vi "Main.vi"(11 "Module Admin":refnum<class "Delacor_lib_QMH_Module Admin.lvclass">) -> ()   [LabVIEW 2022 SP3, in "Motor.lvlib"]
doc: "This template is based off of the Queued Message Handler design pattern and the Queued Message Handler project template that ships with LabVIEW.\n\nThe main difference is that the queue is private to this module and communication between modules is performed via Broadcast and Request events.\n\nRequest events are wrapped in public API methods and are handled in the Event Handling Loop (EHL) of this VI. Any module can register for Broadcast events sent by this module. The EHL generates messages based on user interface actions.\n\nThe Message Handling Loop (MHL) processes messages generated by the EHL, or by other messages. The messages are string values, so new messages can be added easily to the Message Cases case structure in the MHL. Each message cluster can also provide an optional value for Message Data, which is a variant that can be converted to whatever message-specific data is required.\n_____\nBased on DQMH Project Template 7.0.1.1316."
uses:
  Motor.lvlib
  <vilib>/Delacor/Delacor QMH/Libraries/Module Admin_class/Delacor_lib_QMH_Module Admin.lvclass
  Module Data--cluster.ctl
  <vilib>/Delacor/Delacor QMH/Libraries/Message Queue_class/Delacor_lib_QMH_Message Queue.lvclass/Delacor_lib_QMH_Message Queue.ctl
  Stop Argument--cluster.ctl
  <vilib>/Delacor/Delacor QMH/Libraries/Module Admin_class/Delacor_lib_QMH_Module Admin.lvclass/Delacor_lib_QMH_Module Admin.ctl
  Moving Argument--cluster.ctl
  <vilib>/Utility/miscctls.llb/LVPointTypeDef.ctl
  <vilib>/MakerHub/LINX/Private/Type Defs/LINX Ref.ctl
  <vilib>/MakerHub/LINX/Private/Type Defs/Platform.ctl
  <vilib>/MakerHub/LINX/Private/Type Defs/Interface.ctl
  <vilib>/MakerHub/LINX/Private/Device/Type Defs/LINX Device Config.ctl
  <vilib>/MakerHub/LINX/Private/Device/Type Defs/TCP Config.ctl
  <vilib>/MakerHub/LINX/Private/Device/Type Defs/Channels.ctl
  Motorshield/DCMotor/DCMotor.lvclass
  <vilib>/Delacor/Delacor QMH/Libraries/Message Queue_class/Delacor_lib_QMH_Enqueue Message (Single).vi
  <vilib>/Delacor/Delacor QMH/Libraries/Module Admin_class/Delacor_lib_QMH_Get External Launch.vi
  <vilib>/Delacor/Delacor QMH/Libraries/Message Queue_class/Delacor_lib_QMH_Message Queue.lvclass
  <vilib>/MakerHub/LINX/LMH-LINX.lvlib
  <vilib>/MakerHub/LINX/Private/Device/Device.lvlib
  BME680/BME680_dqmh.lvlib
panel:
  out "error out":errorcluster
  out "Status":string
  in  "Simulate MHL Error":bool
  in  "Simulate EHL Error":bool
  # "Other processes communicate with this Module via its Public API (wrappers for its Request Events).\n\nThis Module communicates with other processes via its Broadcast Events.\nAny process that wants to receive these messages can register for this module's Broadcast events."
  # "This template is for the DQMH framework. See the block diagram for more information on how to use this template."
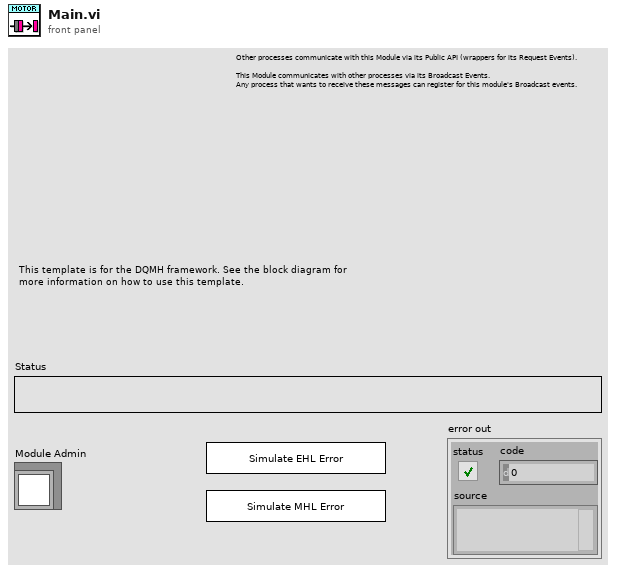
[diagram p1: front panel]
types:
  T1 = typedef "Motor.lvlib/Request Events--cluster.ctl" = cluster{"Stop Module":refnum<user-event>, "Show Panel":refnum<user-event>, "Hide Panel":refnum<user-event>, "Get Module Execution Status":refnum<user-event>, "Show Diagram":refnum<user-event>, "Linx":refnum<user-event>, "Moving":refnum<user-event>}
  T2 = typedef "Motor.lvlib/Module Data--cluster.ctl" = cluster{"Status":string}
  T3 = enum32{"invalid lock state", "Not Locked", "Locked (No Password)", "Password-protected"}
  T4 = typedef "Motor.lvlib/Stop Argument--cluster.ctl" = cluster{"Origin":string, "Exit via Stop Module Req?":bool, "Wait for Module to stop?":bool}
  T5 = typedef "Motor.lvlib/Moving Argument--cluster.ctl" = cluster{"Modul":u8}
  T6 = typedef "LVPointTypeDef.ctl" = cluster{"Horizontal":i16, "Vertical":i16}
  T7 = enum32{"Invalid", "Standard", "Closed", "Hidden", "Minimized", "Maximized"}
  T8 = typedef "LMH-LINX.lvlib/LINX Ref.ctl" = cluster{"IO":T9, "Interface":T10, "LINX Device Config":T11}
  T9 = typedef "LMH-LINX.lvlib/Platform.ctl" = enum16{"Remote", "Local"}
  T10 = typedef "LMH-LINX.lvlib/Interface.ctl" = enum16{"Serial", "TCP"}
  T11 = typedef "LMH-LINX.lvlib/Device.lvlib/LINX Device Config.ctl" = cluster{"Interface":T10, "COM Port":refnum<visa-resource-name>, "TCP Configuration":T12, "Device Family":u8, "Device ID":u8, "Device Name":string, "TCP Ref":refnum<k5>, "Channels":T13}
  T12 = typedef "LMH-LINX.lvlib/Device.lvlib/TCP Config.ctl" = cluster{"IP Address":string, "Port":u16}
  T13 = typedef "LMH-LINX.lvlib/Channels.ctl" = cluster{"DI":u8[], "DO":u8[], "AI":u8[], "AO":u8[], "PWM":u8[], "QE":u8[], "UART":u8[], "I2C 2":u8[], "SPI":u8[], "CAN":u8[], "Servo":u8[], "AI Ref (V)":dbl, "AI Resolution (Bits)":u8, "AO Ref (V)":dbl, "AO Resolution (Bits)":u8}
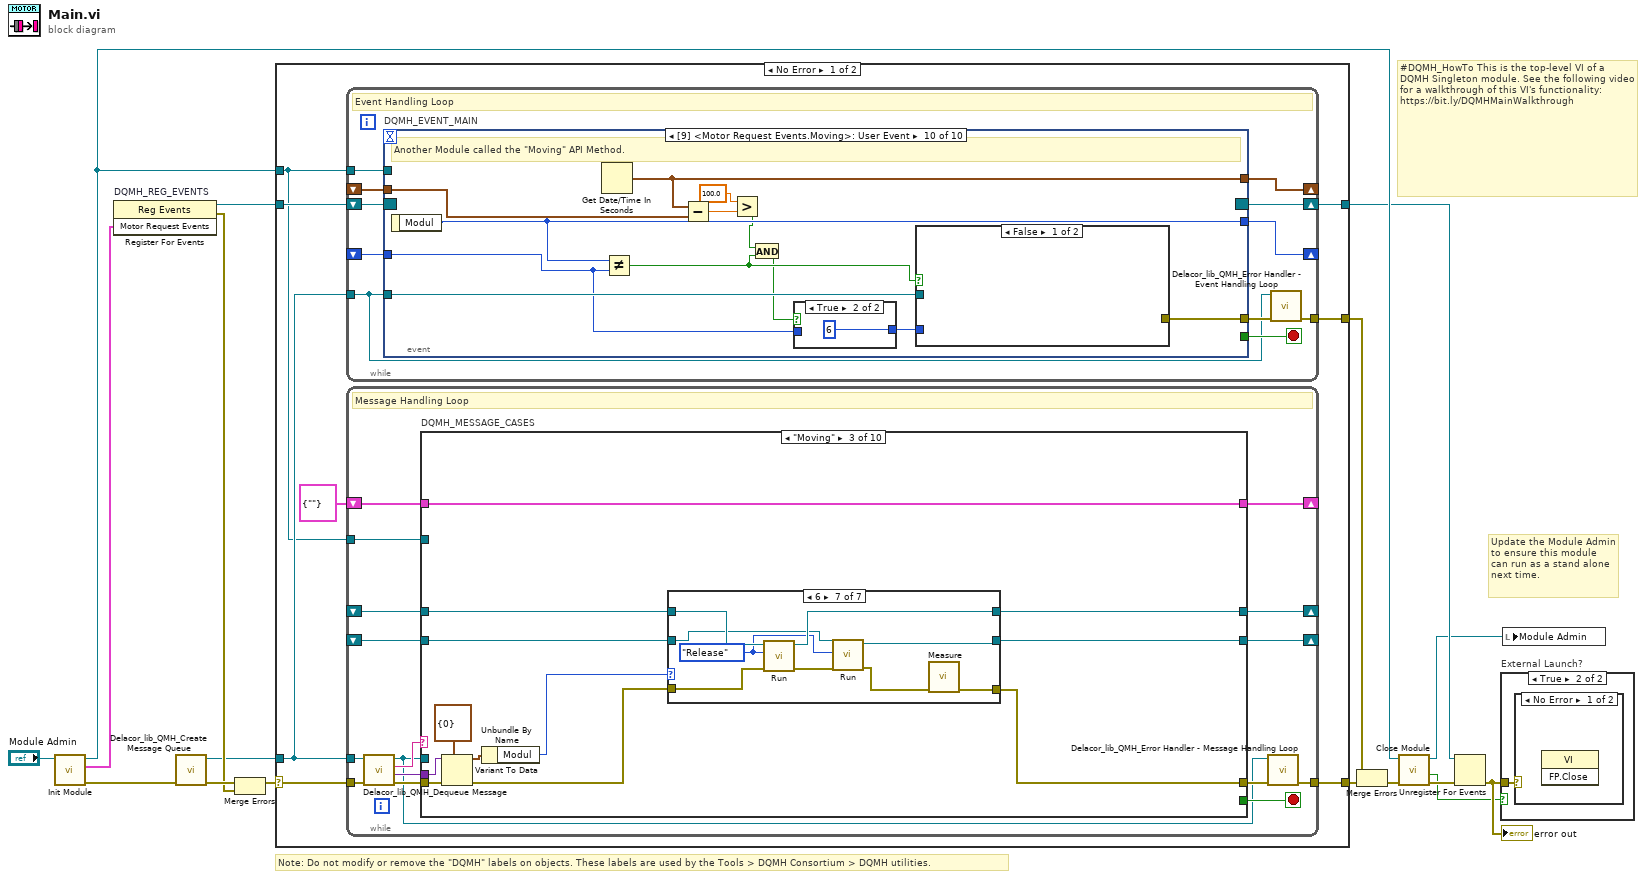
[diagram p0: block diagram]
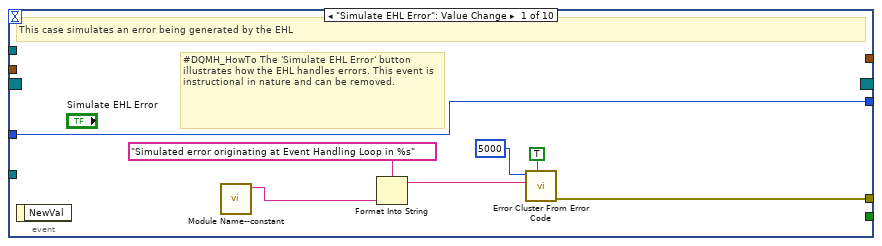
[diagram p2: hidden frame]
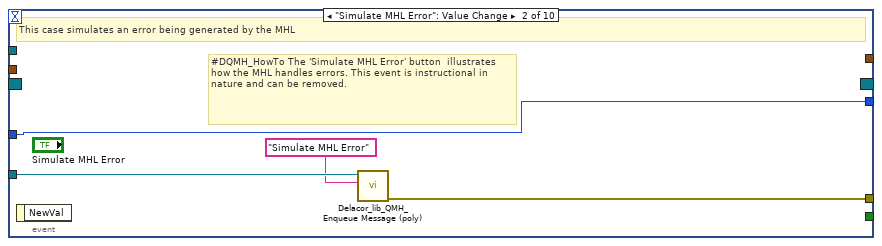
[diagram p3: hidden frame]
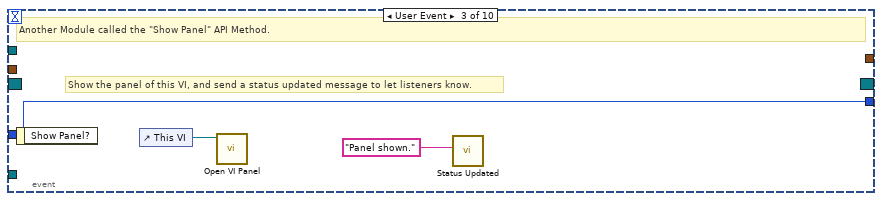
[diagram p4: hidden frame]
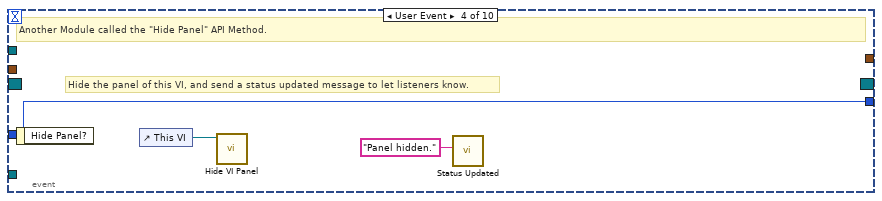
[diagram p5: hidden frame]
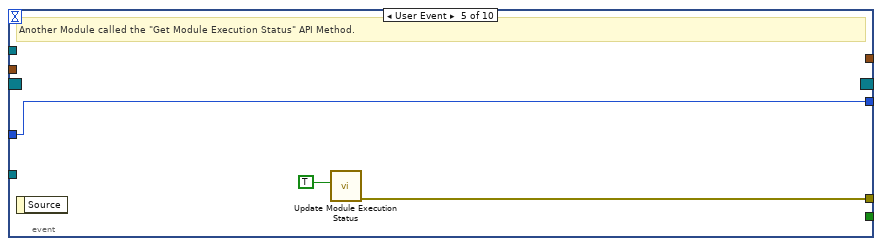
[diagram p6: hidden frame]
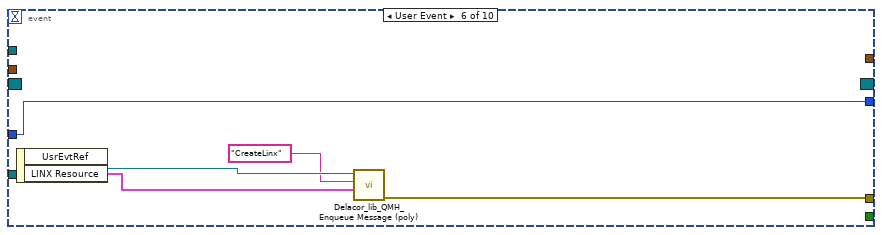
[diagram p7: hidden frame]
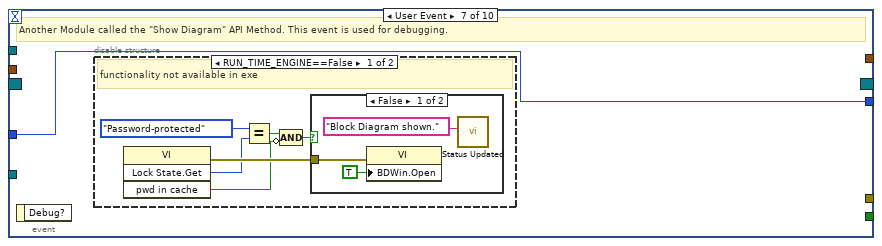
[diagram p8: hidden frame]
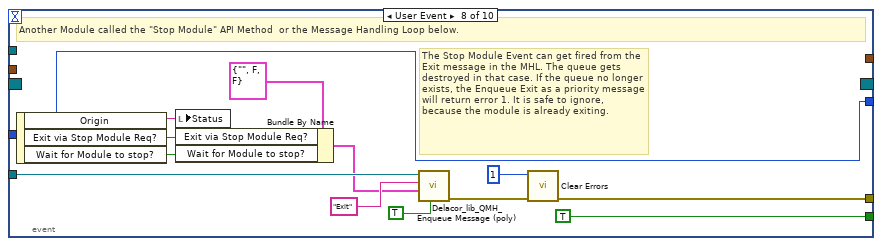
[diagram p11: hidden frame]
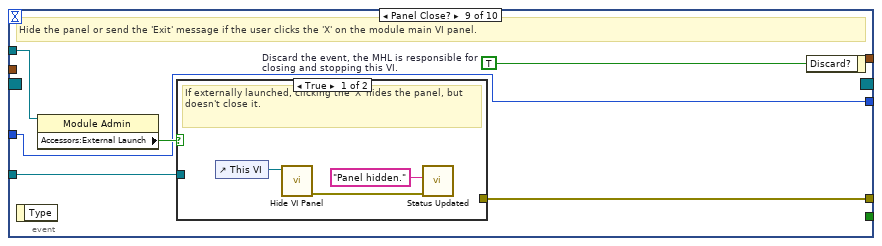
[diagram p12: hidden frame]
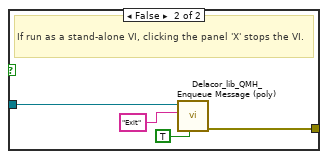
[diagram p13: hidden frame]
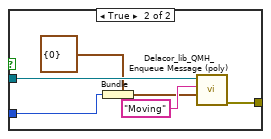
[diagram p15: hidden frame]
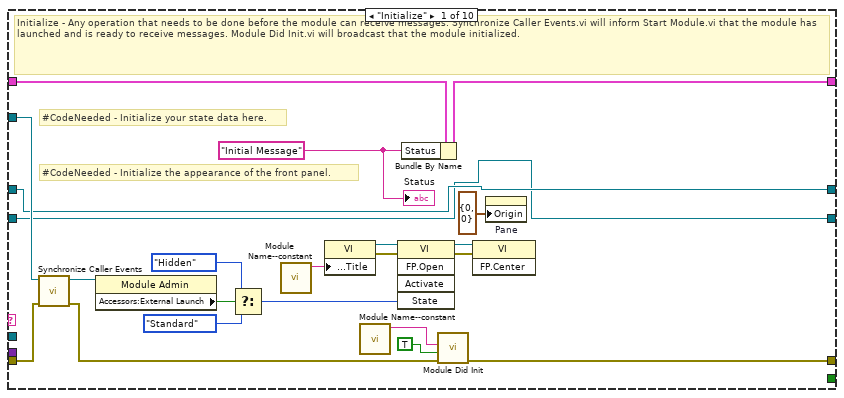
[diagram p16: hidden frame]
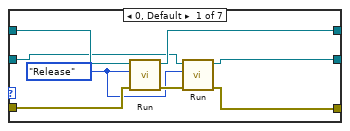
[diagram p18: hidden frame]
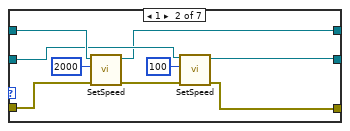
[diagram p19: hidden frame]
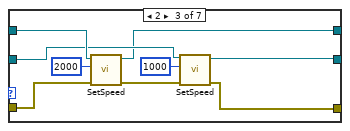
[diagram p20: hidden frame]
diagram:
  # "#DQMH_HowTo This is the top-level VI of a DQMH Singleton module. See the following video for a walkthrough of this VI's functionality: https://bit.ly/DQMHMainWalkthrough"
  # "Note: Do not modify or remove the \"DQMH\" labels on objects. These labels are used by the Tools > DQMH Consortium > DQMH utilities."
  # "Update the Module Admin to ensure this module can run as a stand alone next time."
  n1 = call "Init Module.vi"("Singleton Module Admin in"="Module Admin") -> ("error out"=w16:errorcluster, "Motor Request Events"=w5:T1, "Singleton Module Admin out"=w8:refnum<class "Delacor_lib_QMH_Module Admin.lvclass">)  [unwired: 8 in]
  n2 = register-events "DQMH_REG_EVENTS"(w5) -> (reference out=w6:refnum<event-registration>, error out=w9:errorcluster)  [unwired: 2 in]
  n3 = call <vilib>:"Delacor_lib_QMH_Create Message Queue.vi"("error in"=w16) -> ("error out"=w11:errorcluster, "Message Queue"=w4:refnum<class "Delacor_lib_QMH_Message Queue.lvclass">)  [unwired: 9 in]
  n4 = Merge Errors(w11, w9) -> (w10:errorcluster)
  n5 = case shown="No Error" w10 {
    selector: w10 -> [w23 w333]
    tunnel: [w25 w332] -> w17
    tunnel: [w22 w331] -> w7
    tunnel: w6 -> [w20 w331]
    tunnel: w4 -> [w19 w326]
    tunnel: [w24 _] -> w14
    tunnel: w8 -> [w18 w327]
    frame No Error {
      n6 = while {
        tunnel: w19 -> [w30]
        shift-right: [w33] -> w22
        shift-left: w20 -> [w34]
        tunnel: [w35] -> w24
        tunnel: w18 -> [w31]
        shift-right: [w29] -> _
        shift-left: _ -> [w28]
        shift-right: [w27] -> _
        shift-left: _ -> [w26]
        stop <- w32 stop-if-true
        # "Event Handling Loop"
        n7 = event "DQMH_EVENT_MAIN" shown="[9] <Motor Request Events.Moving>: User Event" {
          selector: w34 -> [_ _ _ _ _ _ _ _ _ _]
          dyn-events: [_ _ _ _ _ _ _ _ _ _] -> w33
          timeout: _ -> [_ _ _ _ _ _ _ _ _ _]
          tunnel: [_ _ _ _ _ _ _ TRUE ("Discard?") _ _] -> w32
          tunnel: w30 -> [_ w46 _ _ _ w60 _ w80 w88 w109]
          tunnel: [w43 w47 _ _ w56 w59 _ w83 w90 w108] -> w36
          tunnel: w31 -> [_ _ _ _ _ _ _ _ w87 _]
          tunnel: [w37 w44 w48 w51 w54 w57 w62 w72 w85 w107] -> w29
          tunnel: w28 -> [w37 w44 w48 w51 w54 w57 w62 w72 w85 w99]
          tunnel: [_ _ _ _ _ _ _ _ _ w106] -> w27
          tunnel: w26 -> [_ _ _ _ _ _ _ _ _ w105]
          event "Simulate EHL Error": Value Change {
            # "#DQMH_HowTo The 'Simulate EHL Error' button  illustrates how the EHL handles errors. This event is instructional in nature and can be removed."
            # "This case simulates an error being generated by the EHL"
            n8 = event-data() -> ()  [unwired: 1 in, 1 out]
            n9 = call "Module Name--constant.vi"() -> ("Module Name"=w40:string)  [unwired: 11 in]
            n10 = Format Into String(format string="Simulated error originating at Event Handling Loop in %s", w40) -> (resulting string=w41:string)  [unwired: 2 in, 1 out]
            n11 = call <vilib>:"Error Cluster From Error Code.vi"("show call chain? (False)"=TRUE, "error message (\"\")"=w41, "error code (0)"=5000) -> ("error out"=w43:errorcluster)  [unwired: 6 in]
          }
          event "Simulate MHL Error": Value Change {
            # "#DQMH_HowTo The 'Simulate MHL Error' button  illustrates how the MHL handles errors. This event is instructional in nature and can be removed."
            # "This case simulates an error being generated by the MHL"
            n12 = event-data() -> ()  [unwired: 1 in, 1 out]
            n13 = call-poly <vilib>:"Delacor_lib_QMH_Enqueue Message (poly).vi"("Message"="Simulate MHL Error", "Message Queue in"=w46) -> ("error out"=w47:errorcluster)  [unwired: 8 in, 1 out]
          }
          event User Event {
            # "Show the panel of this VI, and send a status updated message to let listeners know."
            # "Another Module called the \"Show Panel\" API Method."
            n14 = event-data() -> ()  [unwired: 1 in, 1 out]
            n15 = control-ref of="This VI"() -> (w50:refnum<vi>)
            n16 = call "Open VI Panel.vi"("VI"=w50) -> ()  [unwired: 10 in, 1 out]
            n17 = call "Status Updated.vi"("Status"="Panel shown." ("format string")) -> ()  [unwired: 10 in, 1 out]
          }
          event User Event {
            # "Hide the panel of this VI, and send a status updated message to let listeners know."
            # "Another Module called the \"Hide Panel\" API Method."
            n18 = event-data() -> ()  [unwired: 1 in, 1 out]
            n19 = control-ref of="This VI"() -> (w53:refnum<vi>)
            n20 = call "Hide VI Panel.vi"("VI"=w53) -> ()  [unwired: 10 in, 1 out]
            n21 = call "Status Updated.vi"("Status"="Panel hidden." ("format string")) -> ()  [unwired: 10 in, 1 out]
          }
          event User Event {
            # "Another Module called the \"Get Module Execution Status\" API Method."
            n22 = event-data() -> ()  [unwired: 1 in, 1 out]
            n23 = call "Update Module Execution Status.vi"("Running?"=TRUE) -> ("error out"=w56:errorcluster)  [unwired: 10 in]
          }
          event User Event {
            n24 = event-data() -> ("LINX Resource"=w61:T8)  [unwired: 1 in, 1 out]
            n25 = call-poly <vilib>:"Delacor_lib_QMH_Enqueue Message (poly).vi"("Message Data"=w61, "Message"="CreateLinx", "Message Queue in"=w60) -> ("error out"=w59:errorcluster)  [unwired: 7 in, 1 out]
          }
          event User Event {
            # "Another Module called the \"Show Diagram\" API Method. This event is used for debugging."
            n26 = event-data() -> ()  [unwired: 1 in, 1 out]
            n27 = disable-structure shown="RUN_TIME_ENGINE==False" {
              frame condition #0 (active) {
                # "functionality not available in exe"
                n28 = invoke on="Invoke Node" class="VI" method="Lock State.Get"() -> (error out=w68:errorcluster, "Get Lock State"=w67:T3, "pwd in cache"=w64:bool)  [unwired: 4 in, 1 out]
                n29 = Equal?(x=T3."Password-protected", y=w67) -> (x = y?=w65:bool)
                n30 = Compound Arithmetic op=AND(w65, invert w64) -> (w63:bool)
                n31 = case shown="False" w63 {
                  tunnel: w68 -> [w71 _]
                  frame False {
                    n32 = property on="Property Node" class="VI"(error in=w71, "BDWin.Open"=TRUE ("Block Diagram Window:Open")) -> ()  [unwired: 1 in, 2 out]
                    n33 = call "Status Updated.vi"("Status"="Block Diagram shown." ("format string")) -> ()  [unwired: 10 in, 1 out]
                  }
                  frame True {
                    # "Password-protected VI, and the password is not in the cache. Do not show the diagram."
                  }
                }
              }
              frame condition #1 {
              }
            }
          }
          event User Event {
            # "The Stop Module Event can get fired from the Exit message in the MHL. The queue gets destroyed in that case. If the queue no longer exists, the Enqueue Exit as a priority message will return error 1. It is safe to ignore, because the module is already exiting."
            # "Another Module called the \"Stop Module\" API Method  or the Message Handling Loop below."
            n34 = event-data() -> ("Origin"=w79:string, "Exit via Stop Module Req?"=w75:bool, "Wait for Module to stop?"=w74:bool)  [unwired: 1 in]
            n35 = local write "Status"(w79) -> ()
            n36 = Bundle By Name(cluster=T4 {"Origin"="", "Exit via Stop Module Req?"=FALSE, "Wait for Module to stop?"=FALSE} ("Stop Argument"), "Exit via Stop Module Req?"=w75, "Wait for Module to stop?"=w74) -> (w73:T4)
            n37 = call-poly <vilib>:"Delacor_lib_QMH_Enqueue Message (poly).vi"("Priority Message? (F)"=TRUE, "Message Data"=w73, "Message"="Exit", "Message Queue in"=w80) -> ("error out"=w84:errorcluster)  [unwired: 6 in, 1 out]
            n38 = call <vilib>:"Clear Errors.vi"("error in (no error)"=w84, "specific error code to clear (0: all)"=1) -> ("error out"=w83:errorcluster)  [unwired: 4 in, 1 out]
          }
          event Panel Close? {
            w89 = TRUE  # Discard the event, the MHL is responsible for closing and stopping this VI.
            # "Hide the panel or send the 'Exit' message if the user clicks the 'X' on the module main VI panel."
            n39 = event-data() -> ()  [unwired: 1 in, 1 out]
            n40 = property on="Property Node" class="Module Admin"(reference=w87) -> ("Accessors:External Launch"=w86:bool)  [unwired: 1 in, 2 out]
            n41 = case shown="True" w86 {
              tunnel: w88 -> [_ w96]
              tunnel: [_ w97] -> w90
              frame True {
                # "If externally launched, clicking the 'X' hides the panel, but doesn't close it."
                n42 = control-ref of="This VI"() -> (w93:refnum<vi>)
                n43 = call "Hide VI Panel.vi"("VI"=w93) -> ("error out"=w91:errorcluster)  [unwired: 10 in]
                n44 = call "Status Updated.vi"("error in"=w91, "Status"="Panel hidden." ("format string")) -> ()  [unwired: 9 in, 1 out]
              }
              frame False {
                # "If run as a stand-alone VI, clicking the panel 'X' stops the VI."
                n45 = call-poly <vilib>:"Delacor_lib_QMH_Enqueue Message (poly).vi"("Priority Message? (F)"=TRUE, "Message"="Exit", "Message Queue in"=w96) -> ("error out"=w97:errorcluster)  [unwired: 7 in, 1 out]
              }
            }
            n46 = event-data ("Event Filter Node")("Discard?"=w89) -> ()  [unwired: 1 in, 1 out]
          }
          event User Event {
            # "Another Module called the \"Moving\" API Method."
            n47 = event-data() -> ("Modul"=w107:u8)  [unwired: 1 in]
            n48 = Get Date/Time In Seconds() -> (seconds since 1Jan1904=w106:timestamp)
            n49 = Not Equal?(x=w107, y=w99) -> (x != y?=w102:bool)
            n50 = Subtract(x=w106, y=w105) -> (x-y=w104:dbl)
            n51 = Greater?(x=100.0, y=w104) -> (0:w101:bool)
            n52 = And(x=w101, y=w102) -> (x .and. y?=w100:bool)
            n53 = case shown="True" w100 {
              tunnel: w99 -> [w110 _]
              tunnel: [w110 6] -> w98
              frame False {
              }
              frame True {
              }
            }
            n54 = case shown="False" w102 {
              tunnel: w109 -> [_ w117]
              tunnel: [_ w113] -> w108
              tunnel: w98 -> [_ w112]
              frame False {
              }
              frame True {
                n55 = Bundle(cluster=T5 {"Modul"=0} ("Moving Argument"), "Modul"=w112) -> (w114:T5)
                n56 = call-poly <vilib>:"Delacor_lib_QMH_Enqueue Message (poly).vi"("Message Data"=w114, "Message"="Moving", "Message Queue in"=w117) -> ("error out"=w113:errorcluster)  [unwired: 7 in, 1 out]
              }
            }
          }
        }
        n57 = call-dynamic "Delacor_lib_QMH_Error Handler - Event Handling Loop.vi"("error in"=w36, "Message Queue in"=w30) -> ("dup error in"=w35:errorcluster)  [unwired: 8 in, 1 out]
      }
      n58 = while {
        tunnel: w19 -> [w122]
        shift-right: [w130] -> _
        shift-left: T2 {"Status"=""} ("Data Cluster") -> [w131]
        tunnel: w23 -> [w133]
        tunnel: [w125] -> w25
        tunnel: w18 -> [w126]
        shift-right: [w121] -> _
        shift-left: _ -> [w119]
        shift-right: [w120] -> _
        shift-left: _ -> [w118]
        stop <- w129 stop-if-true
        # "Message Handling Loop"
        n59 = call-dynamic "Delacor_lib_QMH_Dequeue Message.vi"("error in"=w133, "Message Queue in"=w122) -> ("error out"=w132:errorcluster, "Message Data"=w127:variant, "Message"=w128:string, "Message Queue out"=w123:refnum<class "Delacor_lib_QMH_Message Queue.lvclass">)  [unwired: 6 in]
        n60 = case "DQMH_MESSAGE_CASES" shown="\"Moving\"" w128 {
          selector: w128 -> [_ _ _ _ _ _ _ _ _ w321]
          tunnel: w123 -> [_ _ _ _ _ _ _ w283 w307 _]
          tunnel: w132 -> [w153 w159 w171 w256 w262 w266 w277 w290 w313 w324]
          tunnel: [w151 w159 w161 w239 w261 w266 w276 w286 w308 w325] -> w124
          tunnel: w131 -> [w142 w158 w170 w257 w260 w265 w274 w285 w306 w322]
          tunnel: [w141 w158 w170 w257 w260 w265 w274 w285 w306 w322] -> w130
          tunnel: [_ _ _ _ _ _ _ _ w305 _] -> w129
          tunnel: w127 -> [_ _ w169 w255 _ _ _ w284 w304 _]
          tunnel: w126 -> [w143 _ _ _ _ _ _ w282 w299 _]
          tunnel: [w135 w157 w164 w237 w259 w264 w268 w279 w298 w315] -> w121
          tunnel: [w134 w156 w165 w235 w258 w263 w267 w278 w297 w314] -> w120
          tunnel: w119 -> [w135 w157 w163 _ w259 w264 w268 w279 w298 w315]
          tunnel: w118 -> [w134 w156 w166 _ w258 w263 w267 w278 w297 w314]
          frame "Initialize" {
            w137 = "Initial Message" ("Initial Message")
            # "#CodeNeeded - Initialize the appearance of the front panel."
            # "#CodeNeeded - Initialize your state data here."
            # "Initialize - Any operation that needs to be done before the module can receive messages. Synchronize Caller Events.vi will inform Start Module.vi that the module has launched and is ready to receive messages. Module Did Init.vi will broadcast that the module initialized."
            n61 = call "Synchronize Caller Events.vi"("error in"=w153, "Singleton Module Admin in"=w143) -> ("error out"=w152:errorcluster, "Singleton Module Admin out"=w138:refnum<class "Delacor_lib_QMH_Module Admin.lvclass">)  [unwired: 8 in]
            n62 = property on="Property Node" class="Module Admin"(reference=w138) -> ("Accessors:External Launch"=w147:bool)  [unwired: 1 in, 2 out]
            n63 = Select(t=T7."Hidden" ("State"), s=w147, f=T7."Standard" ("State")) -> (s? t:f=w144:T7)
            n64 = call "Module Name--constant.vi"() -> ("Module Name"=w150:string)  [unwired: 11 in]
            n65 = property on="Property Node" class="VI"("Front Panel.Title"=w150) -> (reference out=w149:refnum<vi>, error out=w155:errorcluster)  [unwired: 2 in]
            n66 = call "Module Name--constant.vi"() -> ("Module Name"=w139:string)  [unwired: 11 in]
            n67 = invoke on="Invoke Node" class="VI" method="FP.Open"(reference=w149, error in=w155, "State"=w144) -> (reference out=w148:refnum<vi>, error out=w154:errorcluster)  [unwired: 2 in, 3 out]
            n68 = Bundle By Name(cluster=w142, "Status"=w137) -> (w141:T2)
            n69 = call "Module Did Init.vi"("error in"=w152, "Initialized?"=TRUE, "Origin"=w139) -> ("error out"=w151:errorcluster)  [unwired: 8 in]
            n70 = invoke on="Invoke Node" class="VI" method="FP.Center"(reference=w148, error in=w154) -> ()  [unwired: 1 in, 3 out]
            n71 = property on="Pane" class="Pane"("Origin"=T6 {"Horizontal"=0, "Vertical"=0}) -> ()  [unwired: 2 in, 2 out]
            "Status" <- w137
          }
          frame "---Module Specific---" {
            # "Separator -- The following cases handle messages specific to this Module."
          }
          frame "Moving" {
            n72 = Variant To Data(error in=w171, type=T5 {"Modul"=0} ("Moving Argument"), Variant=w169) -> (data=w167:T5, error out=w162:errorcluster)
            n73 = Unbundle By Name(w167) -> ("Modul"=w160:u8)
            n74 = case shown="6" w160 {
              tunnel: w163 -> [w176 w185 w194 w203 w212 w221 w231]
              tunnel: w166 -> [w174 w184 w193 w202 w211 w220 w229]
              tunnel: w162 -> [w179 w188 w197 w206 w215 w224 w233]
              tunnel: [w177 w186 w195 w204 w213 w222 w225] -> w161
              tunnel: [w175 w183 w192 w201 w210 w219 w230] -> w164
              tunnel: [w173 w182 w191 w200 w209 w218 w228] -> w165
              frame 0, Default {
                w172 = enum16{"Bacward", "Forward", "Release"}."Release" ("Enum")
                n75 = call "Run.vi"("error in (no error)"=w179, "Enum"=w172, "DCMotor in"=w176) -> ("error out"=w178:errorcluster, "DCMotor out"=w175:refnum<class "DCMotor.lvclass">)  [unwired: 7 in]
                n76 = call "Run.vi"("error in (no error)"=w178, "Enum"=w172, "DCMotor in"=w174) -> ("error out"=w177:errorcluster, "DCMotor out"=w173:refnum<class "DCMotor.lvclass">)  [unwired: 7 in]
              }
              frame 1 {
                n77 = call "SetSpeed.vi"("error in (no error)"=w188, "Speed(0..4095)"=u16 2000, "DCMotor in"=w185) -> ("error out"=w187:errorcluster, "DCMotor out"=w183:refnum<class "DCMotor.lvclass">)  [unwired: 7 in]
                n78 = call "SetSpeed.vi"("error in (no error)"=w187, "Speed(0..4095)"=u16 100, "DCMotor in"=w184) -> ("error out"=w186:errorcluster, "DCMotor out"=w182:refnum<class "DCMotor.lvclass">)  [unwired: 7 in]
              }
              frame 2 {
                n79 = call "SetSpeed.vi"("error in (no error)"=w197, "Speed(0..4095)"=u16 2000, "DCMotor in"=w194) -> ("error out"=w196:errorcluster, "DCMotor out"=w192:refnum<class "DCMotor.lvclass">)  [unwired: 7 in]
                n80 = call "SetSpeed.vi"("error in (no error)"=w196, "Speed(0..4095)"=u16 1000, "DCMotor in"=w193) -> ("error out"=w195:errorcluster, "DCMotor out"=w191:refnum<class "DCMotor.lvclass">)  [unwired: 7 in]
              }
              frame 3 {
                n81 = call "SetSpeed.vi"("error in (no error)"=w206, "Speed(0..4095)"=u16 3000, "DCMotor in"=w203) -> ("error out"=w205:errorcluster, "DCMotor out"=w201:refnum<class "DCMotor.lvclass">)  [unwired: 7 in]
                n82 = call "SetSpeed.vi"("error in (no error)"=w205, "Speed(0..4095)"=u16 3000, "DCMotor in"=w202) -> ("error out"=w204:errorcluster, "DCMotor out"=w200:refnum<class "DCMotor.lvclass">)  [unwired: 7 in]
              }
              frame 4 {
                n83 = call "SetSpeed.vi"("error in (no error)"=w215, "Speed(0..4095)"=u16 1000, "DCMotor in"=w212) -> ("error out"=w214:errorcluster, "DCMotor out"=w210:refnum<class "DCMotor.lvclass">)  [unwired: 7 in]
                n84 = call "SetSpeed.vi"("error in (no error)"=w214, "Speed(0..4095)"=u16 2000, "DCMotor in"=w211) -> ("error out"=w213:errorcluster, "DCMotor out"=w209:refnum<class "DCMotor.lvclass">)  [unwired: 7 in]
              }
              frame 5 {
                n85 = call "SetSpeed.vi"("error in (no error)"=w224, "Speed(0..4095)"=u16 1000, "DCMotor in"=w221) -> ("error out"=w223:errorcluster, "DCMotor out"=w219:refnum<class "DCMotor.lvclass">)  [unwired: 7 in]
                n86 = call "SetSpeed.vi"("error in (no error)"=w223, "Speed(0..4095)"=u16 2000, "DCMotor in"=w220) -> ("error out"=w222:errorcluster, "DCMotor out"=w218:refnum<class "DCMotor.lvclass">)  [unwired: 7 in]
              }
              frame 6 {
                w227 = enum16{"Bacward", "Forward", "Release"}."Release" ("Enum")
                n87 = call "Run.vi"("error in (no error)"=w233, "Enum"=w227, "DCMotor in"=w231) -> ("error out"=w232:errorcluster, "DCMotor out"=w230:refnum<class "DCMotor.lvclass">)  [unwired: 7 in]
                n88 = call "Run.vi"("error in (no error)"=w232, "Enum"=w227, "DCMotor in"=w229) -> ("error out"=w226:errorcluster, "DCMotor out"=w228:refnum<class "DCMotor.lvclass">)  [unwired: 7 in]
                n89 = call "Measure.vi"("error in"=w226) -> ("error out"=w225:errorcluster)  [unwired: 10 in]
              }
            }
          }
          frame "CreateLinx" {
            w234 = enum16{"Bacward", "Forward", "Release"}."Forward" ("Enum")
            w250 = u8 61 ("_addr")
            n90 = Variant To Data(error in=w256, type=T8 {"IO"=enum."Remote", "Interface"=enum."Serial", "LINX Device Config"={"Interface"=enum."Serial", "COM Port"="", "TCP Configuration"={"IP Address"="", "Port"=0}, "Device Family"=0, "Device ID"=0, "Device Name"="", "TCP Ref"=refnum, "Channels"={"DI"=[], "DO"=[], "AI"=[], "AO"=[], "PWM"=[], "QE"=[], "UART"=[], "I2C 2"=[], "SPI"=[], "CAN"=[], "Servo"=[], "AI Ref (V)"=0.0, "AI Resolution (Bits)"=0, "AO Ref (V)"=0.0, "AO Resolution (Bits)"=0}}} ("LINX Resource"), Variant=w255) -> (data=w244:T8, error out=w253:errorcluster)
            n91 = call "InitDC.vi"("error in (no error)"=w253, "_addr"=w250, "Motornum"=u8 0, "DCMotor in"=refnum<class "DCMotor.lvclass"> refnum ("Motorshield.lvlib:DCMotor.lvclass")) -> ("error out"=w246:errorcluster, "DCMotor out"=w247:refnum<class "DCMotor.lvclass">)  [unwired: 6 in]
            n92 = call-dynamic "Begin.vi"("error in (no error)"=w246, "LINX Resource"=w244, "DCMotor in"=w247) -> ("error out"=w242:errorcluster, "DCMotor out"=w238:refnum<class "DCMotor.lvclass">)  [unwired: 6 in, 1 out]
            n93 = call "InitDC.vi"("error in (no error)"=w242, "_addr"=w250, "Motornum"=u8 1, "DCMotor in"=refnum<class "DCMotor.lvclass"> refnum ("Motorshield.lvlib:DCMotor.lvclass")) -> ("error out"=w243:errorcluster, "DCMotor out"=w245:refnum<class "DCMotor.lvclass">)  [unwired: 6 in]
            n94 = call-dynamic "Begin.vi"("error in (no error)"=w243, "LINX Resource"=w244, "DCMotor in"=w245) -> ("error out"=w241:errorcluster, "DCMotor out"=w236:refnum<class "DCMotor.lvclass">)  [unwired: 6 in, 1 out]
            n95 = call "Run.vi"("error in (no error)"=w241, "Enum"=w234, "DCMotor in"=w238) -> ("error out"=w240:errorcluster, "DCMotor out"=w237:refnum<class "DCMotor.lvclass">)  [unwired: 7 in]
            n96 = call "Run.vi"("error in (no error)"=w240, "Enum"=w234, "DCMotor in"=w236) -> ("error out"=w239:errorcluster, "DCMotor out"=w235:refnum<class "DCMotor.lvclass">)  [unwired: 7 in]
          }
          frame "---Copy This Frame---" {
            # "Duplicate this frame when creating new messages.  Change this comment in the duplicated frame to describe this message."
            n97 = Merge Errors(w262) -> (w261:errorcluster)
          }
          frame "---Exit and Error Handling---" {
            # "Separator - The following cases handle errors and exit messages."
          }
          frame "Simulate MHL Error" {
            # "#DQMH_HowTo The 'Simulate MHL Error' button  illustrates how the MHL handles errors. This event is instructional in nature and can be removed."
            # "Simulate an error occurring at the MHL"
            n98 = call "Module Name--constant.vi"() -> ("Module Name"=w270:string)  [unwired: 11 in]
            n99 = Format Into String(format string="Simulated error originating at Message Handling Loop in %s", w270) -> (resulting string=w271:string)  [unwired: 2 in, 1 out]
            n100 = call <vilib>:"Error Cluster From Error Code.vi"("show call chain? (False)"=TRUE, "error message (\"\")"=w271, "error code (0)"=5001) -> ("error out"=w275:errorcluster)  [unwired: 6 in]
            n101 = Merge Errors(w277, w275) -> (w276:errorcluster)
          }
          frame "Error" {
            # "#CodeRecommended - If the module is running in standalone mode (External Launch = FALSE), this code will pop up an error dialog and call the 'Exit' message if an error occurs. Add more fine-grained error management here."
            # "Error - Check the error message data and respond accordingly. This message is sent by the \"Error Handler\" VIs at the end of each loop in this application."
            n102 = property on="Property Node" class="Module Admin"(reference=w282) -> ("Accessors:External Launch"=w281:bool)  [unwired: 1 in, 2 out]
            n103 = Variant To Data(error in=w290, type=errorcluster {"status"=FALSE, "code"=0, "source"=""} ("error constant"), Variant=w284) -> (data=w280:errorcluster, error out=w288:errorcluster)
            n104 = local write "error out"(w280) -> ()
            n105 = call "Error Reported.vi"("Error"=w280) -> ()  [unwired: 10 in, 1 out]
            n106 = case shown="False" w281 {
              tunnel: [w295 _] -> w287
              tunnel: w283 -> [w293 _]
              tunnel: w280 -> [w294 _]
              frame False {
                n107 = disable-structure shown="Default" {
                  disable-tunnel: w294 -> [w296 _]
                  frame condition #0 (active) {
                    # "If the module is running standalone, then pop up an error dialog and call the \"Exit\" message."
                    n108 = call <vilib>:"Simple Error Handler.vi"("error in (no error)"=w296) -> ()  [unwired: 4 in, 5 out]
                  }
                  frame condition #1 {
                    # "To prevent the Simple Error Handler VI from being loaded (e.g. when deploying to a Real-Time target), add the Conditional Disable Symbol \"DQMH_Disable_SEH\" to your project and set it to TRUE."
                  }
                }
                n109 = call-poly <vilib>:"Delacor_lib_QMH_Enqueue Message (poly).vi"("Priority Message? (F)"=TRUE, "Message"="Exit", "Message Queue in"=w293) -> ("error out"=w295:errorcluster)  [unwired: 7 in, 1 out]
              }
              frame True {
                # "If the module was launched externally, calling the Error Reported broadcast VI is the only action performed by the \"Error\" message. The module's caller can then process the error appropriately."
              }
            }
            n110 = Merge Errors(w288, w287) -> (w286:errorcluster)
          }
          frame "Exit" {
            w303 = 91  # 91: not all Exit messages will have an argument
            w305 = TRUE  # Stop the VI
            # "Release the message queue reference"
            # "#CodeNeeded - Add any required cleanup code here."
            # "Exit - Exit the application."
            n111 = Variant To Data(error in=w313, type=T4 {"Origin"="", "Exit via Stop Module Req?"=FALSE, "Wait for Module to stop?"=FALSE} ("Stop Argument"), Variant=w304) -> (data=w301:T4, error out=w310:errorcluster)
            n112 = call <vilib>:"Clear Errors.vi"("error in (no error)"=w310, "specific error code to clear (0: all)"=w303) -> ("error out"=w312:errorcluster)  [unwired: 4 in, 1 out]
            n113 = control-ref of="This VI"() -> (w300:refnum<vi>)
            n114 = call-dynamic "Delacor_lib_QMH_Release Message Queue.vi"("error in"=w312, "Message Queue"=w307) -> ("error out"=w311:errorcluster)  [unwired: 9 in]
            n115 = call "Handle Exit.vi"("Stop Argument"=w301, "Admin in"=w299, "VI reference"=w300) -> ("error out"=w309:errorcluster)  [unwired: 7 in, 1 out]
            n116 = Merge Errors(w311, w309) -> (w308:errorcluster)
            n117 = call "Error Reported.vi"("Error"=w308) -> ()  [unwired: 10 in, 1 out]
          }
          frame Default {
            # "'Default' case only runs if there is a message that isn't defined in any of the other cases.  Output a programming error."
            n118 = call "Module Name--constant.vi"() -> ("Module Name"=w320:string)  [unwired: 11 in]
            n119 = Format Into String(format string="The invalid message string \"%s\" was received in the Message Handling Loop for module \"%s\".", w321, w320) -> (resulting string=w316:string)  [unwired: 2 in, 1 out]
            n120 = call <vilib>:"Error Cluster From Error Code.vi"("show call chain? (False)"=TRUE, "error message (\"\")"=w316, "error code (0)"=1) -> ("error out"=w323:errorcluster)  [unwired: 6 in]
            n121 = Merge Errors(w324, w323) -> (w325:errorcluster)
          }
        }
        n122 = call-dynamic "Delacor_lib_QMH_Error Handler - Message Handling Loop.vi"("error in"=w124, "Message Queue in"=w123) -> ("dup error in"=w125:errorcluster)  [unwired: 8 in, 1 out]
      }
    }
    frame Error {
      # "Synchronize Caller Events.vi will inform Start Module.vi that the module has launched and will let the code calling Start Module.vi register for broadcasts and would permit the caller receive the broadcast that an error occurred at launch time."
      n123 = call-dynamic "Delacor_lib_QMH_Release Message Queue.vi"("error in"=w333, "Message Queue"=w326) -> ("error out"=w332:errorcluster)  [unwired: 9 in]
      n124 = call "Synchronize Caller Events.vi"("Singleton Module Admin in"=w327) -> ("error out"=w334:errorcluster)  [unwired: 9 in, 1 out]
      n125 = call "Module Name--constant.vi"() -> ("Module Name"=w330:string)  [unwired: 11 in]
      n126 = Format Into String(format string="An error occurred during initialization. %s is no longer running.", w330) -> (resulting string=w328:string)  [unwired: 2 in, 1 out]
      n127 = Merge Errors(w332, w334) -> (w335:errorcluster)
      n128 = call "Error Reported.vi"("Additional Information"=w328, "Error"=w335) -> ()  [unwired: 9 in, 1 out]
    }
  }
  n129 = Merge Errors(w14, w17) -> (w13:errorcluster)
  n130 = call "Close Module.vi"("error in"=w13, "Module Admin in"=w8) -> ("error out"=w15:errorcluster, "External Launch"=w1:bool, "Module Admin out"=w2:refnum<class "Delacor_lib_QMH_Module Admin.lvclass">)  [unwired: 7 in]
  n131 = Unregister For Events(event registration refnum=w7, error in=w15) -> (error out=w12:errorcluster)
  "error out" <- w12
  n132 = case "External Launch?" shown="True" w1 {
    tunnel: w12 -> [_ w336]
    frame False {
    }
    frame True {
      n133 = case shown="No Error" w336 {
        frame No Error {
          n134 = invoke on="Invoke Node" class="VI" method="FP.Close"() -> ()  [unwired: 3 in, 3 out]
        }
        frame Error {
          n135 = invoke on="Invoke Node" class="VI" method="FP.Open"("Activate"=TRUE ("Activate?")) -> ()  [unwired: 4 in, 5 out]
        }
      }
    }
  }
  n136 = local write "Module Admin"(w2) -> ()
